vi "Stream Stop.vi"(8 "error in (no error)":errorcluster, 11 "DAQ_msgHandler StreamTypeDef":T1) -> (0 "error out":errorcluster, 3 "DAQ_msgHandler StreamTypeDef 2":T1)   [LabVIEW 2024]
doc: "This VI uses the TDMS Write function to write data to a TDMS file."
uses:
  CTRsample/Control/streamIO_states.ctl
  controls/DAQ_msgHandler StreamTypeDef.ctl
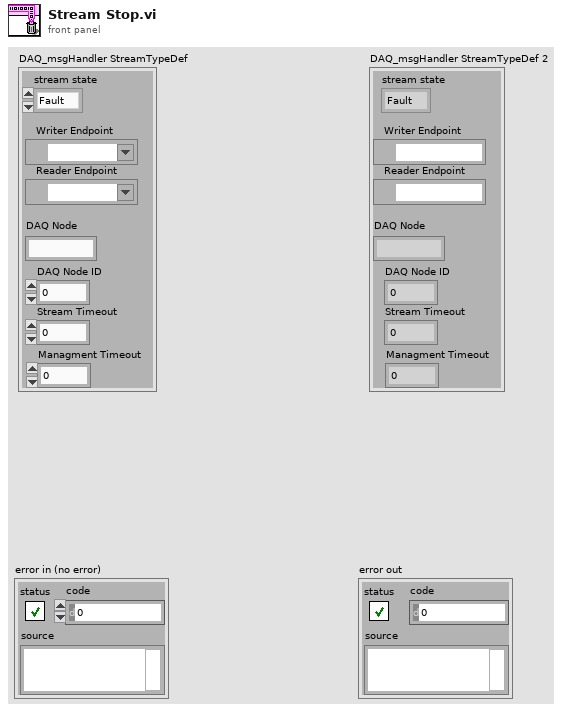
[diagram p1: front panel]
types:
  T1 = typedef "DAQ_msgHandler StreamTypeDef.ctl" = cluster{"stream state":T2, "DAQ Node":string, "DAQ Node ID":i32, "Writer Endpoint":refnum<k21>, "Reader Endpoint":refnum<k21>, "Stream Timeout":dbl, "Managment Timeout":dbl}
  T2 = typedef "streamIO_states.ctl" = enum16{"Fault", "Initilize", "Stream", "Close"}
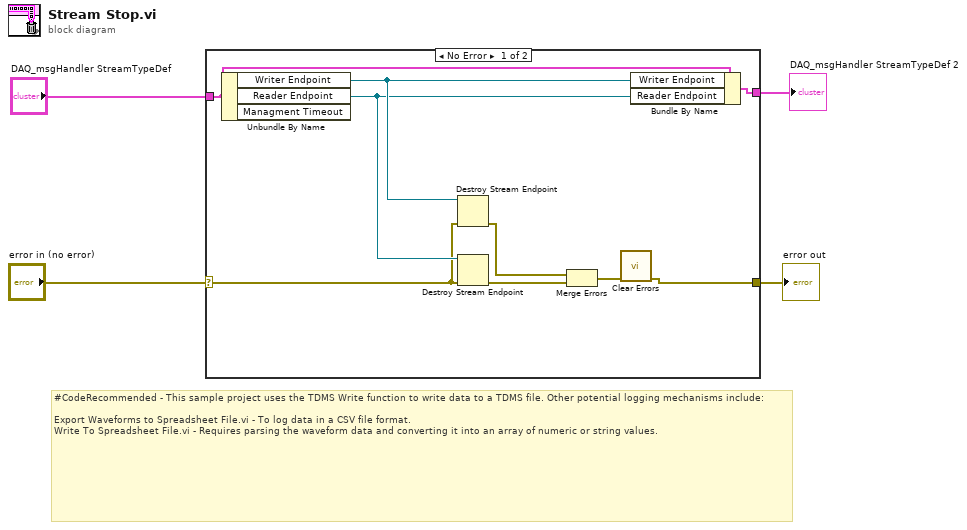
[diagram p0: block diagram]
diagram:
  # "#CodeRecommended - This sample project uses the TDMS Write function to write data to a TDMS file. Other potential logging mechanisms include:\n\nExport Waveforms to Spreadsheet File.vi - To log data in a CSV file format.\nWrite To Spreadsheet File.vi - Requires parsing the waveform data and converting it into an array of numeric or string values."
  n1 = case shown="No Error" "error in (no error)" {
    selector: "error in (no error)" -> [w9 w15]
    tunnel: [w5 w15] -> w4
    tunnel: "DAQ_msgHandler StreamTypeDef" -> [w13 w14]
    tunnel: [w12 w14] -> w1
    frame No Error {
      n2 = Unbundle By Name(w13) -> ("Writer Endpoint"=w11:refnum<k21>, "Reader Endpoint"=w10:refnum<k21>)  [unwired: 1 out]
      n3 = Destroy Stream Endpoint(8:w9, 11:w11) -> (0:w8:errorcluster)
      n4 = Destroy Stream Endpoint(8:w9, 11:w10) -> (0:w7:errorcluster)
      n5 = Merge Errors(w8, w7) -> (w6:errorcluster)
      n6 = call <vilib>:"Clear Errors.vi"("error in (no error)"=w6) -> ("error out"=w5:errorcluster)  [unwired: 5 in, 1 out]
      n7 = Bundle By Name(cluster=w13, "Writer Endpoint"=w11, "Reader Endpoint"=w10) -> (w12:T1)
    }
    frame Error {
    }
  }
  "error out" <- w4
  "DAQ_msgHandler StreamTypeDef 2" <- w1
